vi "Read Trace (Swept SA).vi"(8 "error in (no error)":errorcluster, 9 "Trace Name (1: Trace 1)":i32(ring)=1 items=["Trace 1"=1, "Trace 2"=2, "Trace 3"=3, "Trace 4"=4], 10 "Timeout (10000 ms)":i32=10000 format="%.0g", 11 "VISA resource name":refnum<visa-resource-name>) -> (0 "error out":errorcluster, 2 "Trace Waveform":cluster{"X Array":dbl[], "Y Array":dbl[]}(graph), 3 "VISA resource name out":refnum<visa-resource-name>)   [LabVIEW 2014, in "Agilent MXA Series.lvlib"]
doc: "Reads the trace from the spectrum analyzer(Swept SA)."
uses:
  Agilent MXA Series.lvlib
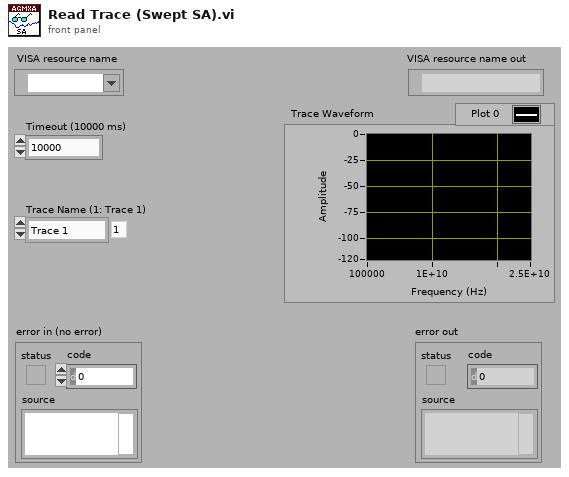
[diagram p1: front panel]
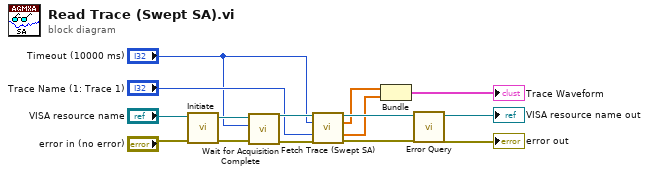
[diagram p0: block diagram]
diagram:
  n1 = call "Initiate.vi"("error in (no error)"="error in (no error)", "VISA resource name"="VISA resource name") -> ("error out"=w12:errorcluster, "VISA resource name out"=w13:refnum<visa-resource-name>)  [unwired: 8 in]
  n2 = call "Wait for Acquisition Complete.vi"("error in (no error)"=w12, "Maximum Time (10000)"="Timeout (10000 ms)", "VISA resource name"=w13) -> ("error out"=w10:errorcluster, "VISA resource name out"=w11:refnum<visa-resource-name>)  [unwired: 7 in]
  n3 = call "Fetch Trace (Swept SA).vi"("VISA resource name"=w11, "Timeout (10000 ms)"="Timeout (10000 ms)", "Trace Name (1: Trace 1)"="Trace Name (1: Trace 1)", "error in (no error)"=w10) -> ("VISA resource name out"=w8:refnum<visa-resource-name>, "X Array"=w4:dbl[], "Y Array"=w3:dbl[], "error out"=w7:errorcluster)  [unwired: 8 in]
  n4 = Bundle("X Array"=w4, "Y Array"=w3) -> (→"Trace Waveform":cluster{"X Array":dbl[], "Y Array":dbl[]})  [unwired: 1 in]
  n5 = call "Error Query.vi"("error in (no error)"=w7, "VISA resource name"=w8) -> ("error out"=→"error out":errorcluster, "VISA resource name out"=→"VISA resource name out":refnum<visa-resource-name>)  [unwired: 6 in, 2 out]
